vi "C2F CONVERTER using sub vi.vi"() -> ()   [LabVIEW 2018]
panel:
  out "High temp":bool
  in  "?":bool
  out "?":string
  out "FARENHEIT (DIGITAL)":dbl
  out "FARENHEIT":dbl(slide) scale=0.0..100.0
  in  "CELSIUS":dbl
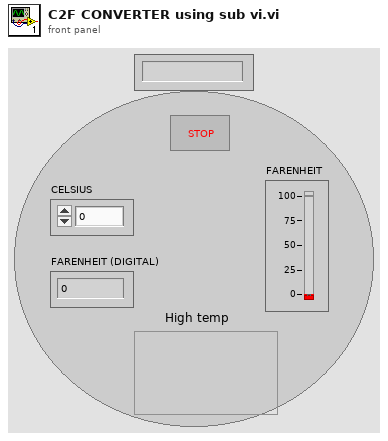
[diagram p1: front panel]
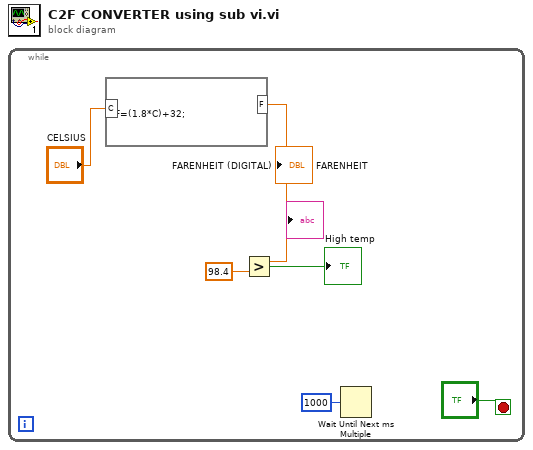
[diagram p0: block diagram]
diagram:
  n1 = while {
    stop <- "?" stop-if-true
    n2 = formula code="F=(1.8*C)+32;"("C"="CELSIUS") -> ("F"=w1:dbl)
    "FARENHEIT" <- w1
    "FARENHEIT (DIGITAL)" <- w1
    n3 = Greater?(x=w1, y=98.4) -> (0:→"High temp":bool)
    n4 = Wait Until Next ms Multiple(millisecond multiple=u32 1000) -> ()  [unwired: 1 out]
  }
